vi "roll.vi"() -> ()   [LabVIEW 2009]
uses:
  <vilib>/rvi/FXPMathLib/FxpAtan2/XNode/nifxpmath_Atan2.xnode
  <vilib>/rvi/FXPMathLib/FxpAtan2/subVIs/nifxpmath_Atan2_SimConfig.ctl
  <vilib>/rvi/FXPMathLib/FxpAtan2/simVIs/DllFxpAtan2Temp_sub.vi
panel:
  out "roll":fxp<+/-,16,2> format="%.15g"
  in  "q3":i16
  in  "q2":i16
  in  "q1":i16
  in  "q0":i16
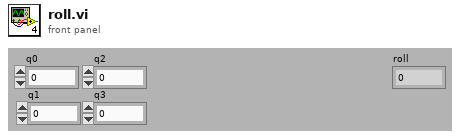
[diagram p1: front panel]
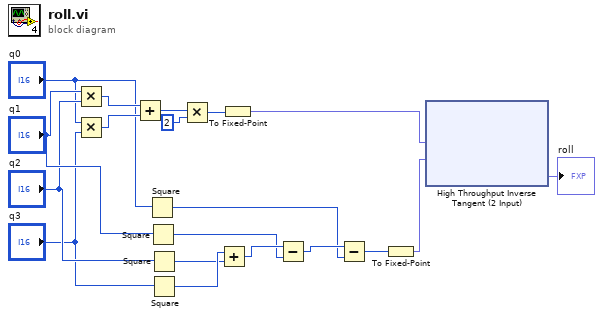
[diagram p0: block diagram]
diagram:
  n1 = Multiply(x="q1", y="q2") -> (x*y=w19:i16)
  n2 = Multiply(x="q0", y="q3") -> (x*y=w18:i16)
  n3 = Add(x=w19, y=w18) -> (x+y=w17:i16)
  n4 = Square(x="q0") -> (x^2=w10:i16)
  n5 = Square(x="q1") -> (x^2=w12:i16)
  n6 = Square(x="q2") -> (x^2=w13:i16)
  n7 = Square(x="q3") -> (x^2=w14:i16)
  n8 = Multiply(x=w17, y=i16 2) -> (x*y=w7:i16)
  n9 = Add(x=w14, y=w13) -> (x+y=w15:i16)
  n10 = To Fixed-Point(number=w7) -> (fixed-point=w6:fxp<+/-,16,16>)  [unwired: 1 in]
  n11 = Subtract(x=w15, y=w12) -> (x-y=w11:i16)
  n12 = Subtract(x=w11, y=w10) -> (x-y=w9:i16)
  n13 = To Fixed-Point(number=w9) -> (fixed-point=w8:fxp<+/-,16,16>)  [unwired: 1 in]
  n14 = xnode "High Throughput Inverse Tangent (2 Input)"("y"=w6, "x"=w8) -> ("atan2(y,x) (pi)"=→"roll":fxp<+/-,16,2>)
